vi "Configure Trigger1.vi"(6 "Manual Trigger Delay (1 s)":dbl=1.0, 8 "error in (no error)":errorcluster, 9 "Auto Delay (T:Enable)":bool=TRUE, 10 "Trigger Source (0: Immediate)":i32(ring) items=["Immediate", "Software (Bus)", "External"], 11 "VISA resource name":refnum<visa-resource-name>) -> (0 "error out":errorcluster, 3 "VISA resource name out":refnum<visa-resource-name>)   [LabVIEW 2015, in "Agilent 3446X Series1.lvlib"]
doc: "Configures the trigger settings on the instrument.\n\n<B>Note:</B> Use this VI only with other low-level VIs. The high-level VIs automatically incorporate this functionality."
uses:
  Agilent 3446X Series1.lvlib
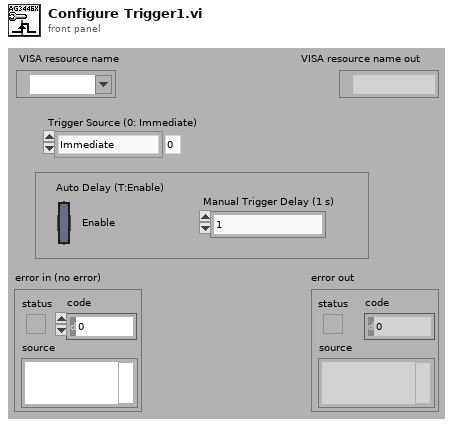
[diagram p1: front panel]
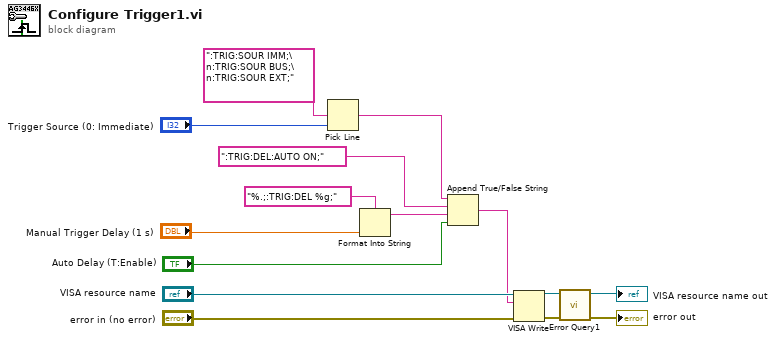
[diagram p0: block diagram]
diagram:
  n1 = Pick Line(multi-line string=":TRIG:SOUR IMM;\n:TRIG:SOUR BUS;\n:TRIG:SOUR EXT;" ("Trigger Source"), line index="Trigger Source (0: Immediate)") -> (output string=w6:string)  [unwired: 1 out]
  n2 = Format Into String(format string="%.;:TRIG:DEL %g;" ("Manual Trigger Delay"), "Manual Trigger Delay (1 s)") -> (resulting string=w7:string)  [unwired: 2 in, 1 out]
  n3 = Append True/False String(1:"Auto Delay (T:Enable)", 2:w7, 3:":TRIG:DEL:AUTO ON;" ("Enable Auto Delay"), 4:w6) -> (0:w5:string)
  n4 = VISA Write(VISA resource name="VISA resource name", write buffer=w5, error in (no error)="error in (no error)") -> (VISA resource name out=w4:refnum<visa-resource-name>, error out=w3:errorcluster)  [unwired: 1 out]
  n5 = call "Error Query1.vi"("error in (no error)"=w3, "VISA resource name"=w4) -> ("error out"=→"error out":errorcluster, "VISA resource name out"=→"VISA resource name out":refnum<visa-resource-name>)  [unwired: 8 out]
